vi "SimpleInitiate.vi"(2 "error in (no error)":errorcluster, 3 "VISA resource name":refnum<visa-resource-name>) -> (0 "error out":errorcluster, 1 "VISA resource name out":refnum<visa-resource-name>)   [LabVIEW 2013]
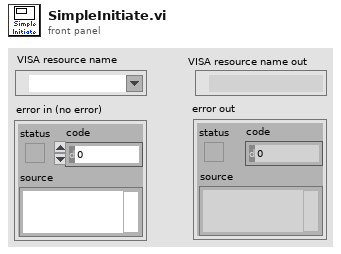
[diagram p1: front panel]
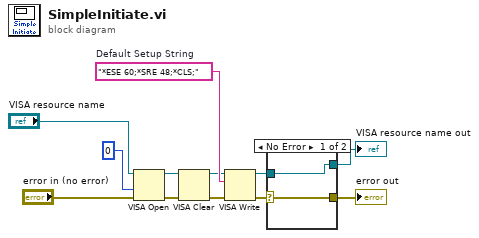
[diagram p0: block diagram]
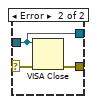
[diagram p2: hidden frame]
diagram:
  w7 = "*ESE 60;*SRE 48;*CLS;"  # Default Setup String
  n1 = VISA Open(access mode=u32 0, error in (no error)="error in (no error)", VISA resource name="VISA resource name") -> (VISA resource name=w9:refnum<visa-resource-name>, error out=w8:errorcluster)  [unwired: 2 in]
  n2 = VISA Clear(VISA resource name=w9, error in (no error)=w8) -> (VISA resource name out=w6:refnum<visa-resource-name>, error out=w5:errorcluster)
  n3 = VISA Write(VISA resource name=w6, write buffer=w7, error in (no error)=w5) -> (VISA resource name out=w3:refnum<visa-resource-name>, error out=w4:errorcluster)  [unwired: 1 out]
  n4 = case shown="No Error" w4 {
    selector: w4 -> [w13 w17]
    tunnel: w3 -> [w14 w15]
    tunnel: [w14 w15] -> w2
    tunnel: [w13 w16] -> w1
    frame No Error {
    }
    frame Error {
      n5 = VISA Close(VISA resource name=w15, error in (no error)=w17) -> (error out=w16:errorcluster)
    }
  }
  "VISA resource name out" <- w2
  "error out" <- w1
